vi "String-to-IMAQdxAttribute.vi"(3 "error in":errorcluster, 5 "IMAQdx-string":string="CameraAttributes::ImageFormatControl::PixelFormat ,Enum ,1,1, 17563719;Mono 8=17301505 ;Mono 12=17825797 ;Mono 12p=17563719 ") -> (0 "error out":errorcluster, 1 "output 2":string, 2 "Attribute Information 2":T2)   [LabVIEW 2011]
uses:
  <vilib>/vision/driver/IMAQdx.llb/IMAQdx Attribute Type.ctl
  <vilib>/vision/driver/NI_Vision_Acquisition_Software.lvlib
panel:
  # "Format: Name, Type[U32,I64,DBL,String,Enum,Bool,Command], Readable[0,1], Wrietable[0,1], Value"
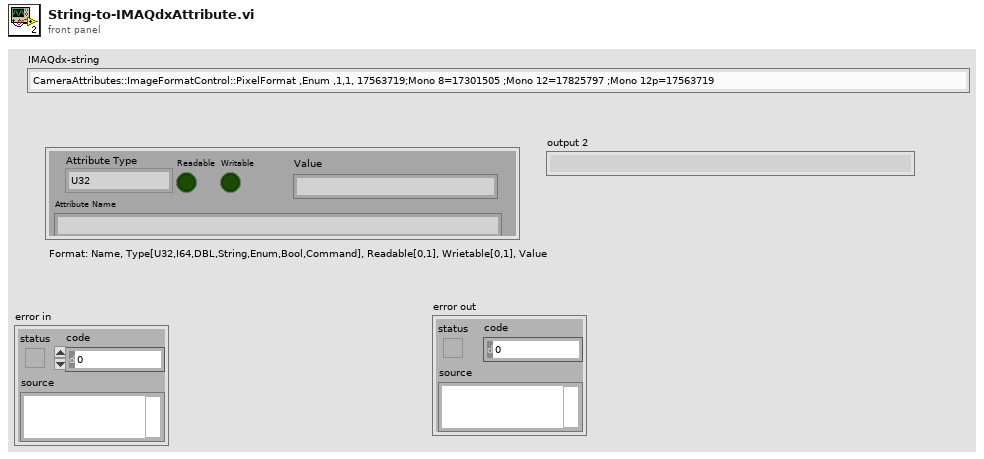
[diagram p1: front panel]
types:
  T1 = typedef "NI_Vision_Acquisition_Software.lvlib/IMAQdx Attribute Type.ctl" = enum32{"U32", "I64", "DBL", "String", "Enum", "Bool", "Command"}
  T2 = cluster{"Attribute Type":T1, "Readable":bool, "Writable":bool, "Attribute Name":string, "Value":string}
  T3 = cluster{"index of element":i32, bool, bool, "default value 1":string, "default value 5":string}
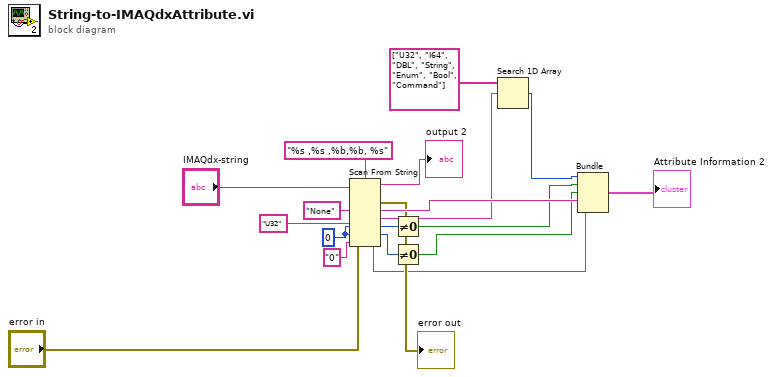
[diagram p0: block diagram]
diagram:
  w9 = 0 ("default value 3")
  n1 = Scan From String(format string="%s ,%s ,%b,%b, %s", input string="IMAQdx-string", error in="error in", default 1="None" ("default value 1"), default 2="U32" ("default value 2"), default 3=w9, default 4=w9, default 5="0" ("default value 5")) -> (remaining string=→"output 2":string, error out=→"error out":errorcluster, output 1=w18:string, output 2=w6:string, output 3=w15:i32, output 4=w13:i32, output 5=w3:string)  [unwired: 1 in, 1 out]
  n2 = Not Equal To 0?(x=w15) -> (x != 0?=w14:bool)
  n3 = Not Equal To 0?(x=w13) -> (x != 0?=w12:bool)
  n4 = Search 1D Array(1D array=string[] ["U32", "I64", "DBL", "String", "Enum", "Bool", "Command"] ("Strings []"), element=w6) -> (index of element=w5:i32)  [unwired: 1 in]
  n5 = Bundle("index of element"=w5, w14, w12, "default value 1"=w18, "default value 5"=w3) -> (→"Attribute Information 2":T3)  [unwired: 1 in]
